vi "GetCtrlInd.vi"(0 "Agents VI Path":path, 1 "error in":errorcluster) -> (2 "Agent VI indicators":cluster{"Name":string, "Variant Data":variant}[](array[cluster]), 3 "Agent VI controls":cluster{"Name":string, "Variant Data":variant}[](array[cluster]), 4 "error out":errorcluster)   [LabVIEW 2009, in "HGF_VisitorGenerator.lvlib"]
doc: "Read indicators and controls linked to the conPane of a VI"
uses:
  HGF_VisitorGenerator.lvlib
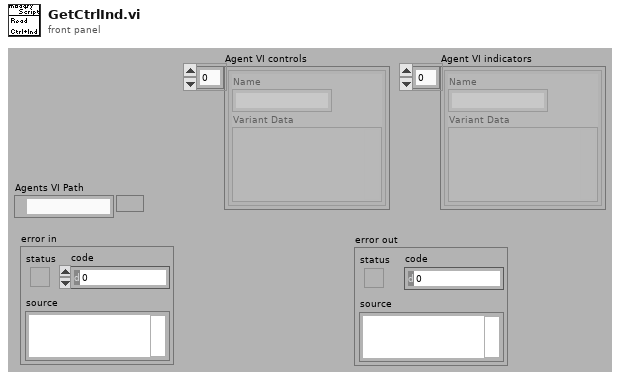
[diagram p1: front panel]
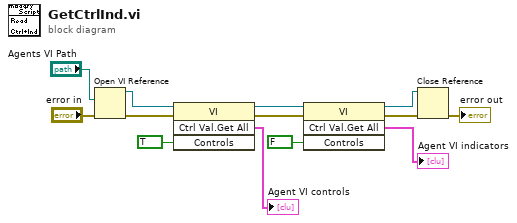
[diagram p0: block diagram]
diagram:
  n1 = Open VI Reference(vi path="Agents VI Path", error in (no error)="error in") -> (vi reference=w1:refnum<vi>, error out=w5:errorcluster)  [unwired: 4 in]
  n2 = invoke class="VI" method="Ctrl Val.Get All"(reference=w1, error in=w5, "Controls"=TRUE) -> (reference out=w3:refnum<vi>, error out=w6:errorcluster, "Get All Control Values Variant"=→"Agent VI controls":cluster{"Name":string, "Variant Data":variant}[])  [unwired: 1 in, 1 out]
  n3 = invoke class="VI" method="Ctrl Val.Get All"(reference=w3, error in=w6, "Controls"=FALSE) -> (reference out=w4:refnum<vi>, error out=w7:errorcluster, "Get All Control Values Variant"=→"Agent VI indicators":cluster{"Name":string, "Variant Data":variant}[])  [unwired: 1 in, 1 out]
  n4 = Close Reference(reference=w4, error in (no error)=w7) -> (error out=→"error out":errorcluster)
